vi "CSM - Convert Argument to Error.vi"(4 "Argument":string) -> (1 "error":errorcluster)   [LabVIEW 2020, in "Communicable State Machine.lvlib"]
uses:
  Communicable State Machine.lvlib
  CSM - Keywords.vi
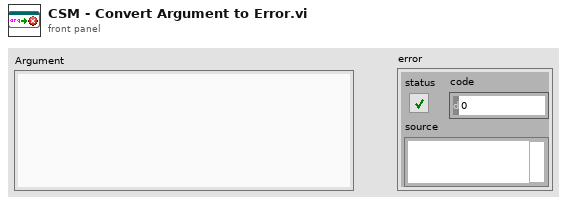
[diagram p1: front panel]
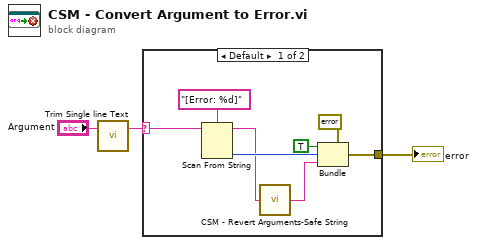
[diagram p0: block diagram]
diagram:
  n1 = call "Trim Single line Text.vi"("single-line text"="Argument") -> ("trimed text"=w2:string)  [unwired: 2 in]
  n2 = case shown="Default" w2 {
    selector: w2 -> [w6 _]
    tunnel: [w7 _] -> w1
    frame Default {
      n3 = Scan From String(format string="[Error: %d]", input string=w6) -> (remaining string=w4:string, output 1=w9:i32)  [unwired: 3 in, 2 out]
      n4 = call "CSM - Revert Arguments-Safe String.vi"("Safe Argurment String"=w4) -> ("Origin Argurment String"=w5:string)  [unwired: 8 in]
      n5 = Bundle(cluster=errorcluster {"status"=TRUE, "code"=0, "source"=""} ("error in (no error)"), "status"=TRUE, "code"=w9, "source"=w5) -> (w7:errorcluster)
    }
    frame "" {
    }
  }
  "error" <- w1
